vi "TEST - Remove Typedefs from Variant.vi"(8 "error in (no error)":errorcluster) -> (0 "error out":errorcluster, 2 "pass":bool)   [LabVIEW 2020, in "test_openg_variant.lvlib"]
uses:
  test_openg_variant.lvlib
  <userlib>/_OpenG.lib/error/error.llb/openg_error.lvlib
  source/library/openg_variant.lvlib
  Type Def.ctl
panel:
  out "Failures":T1(array[cluster])
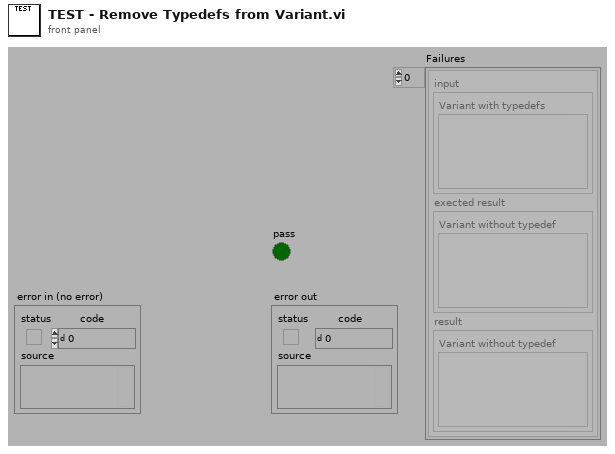
[diagram p1: front panel]
types:
  T1 = cluster{"input":cluster{"Variant with typedefs":variant}, "exected result":cluster{"Variant without typedef":variant}, "result":cluster{"Variant without typedef":variant}}[]
  T2 = typedef "test_openg_variant.lvlib/Type Def.ctl" = dbl
  T3 = cluster{"input":cluster{"Variant with typedefs":variant}, "exected result":cluster{"Variant without typedef":variant}, "result":cluster{"Variant without typedef":variant}}
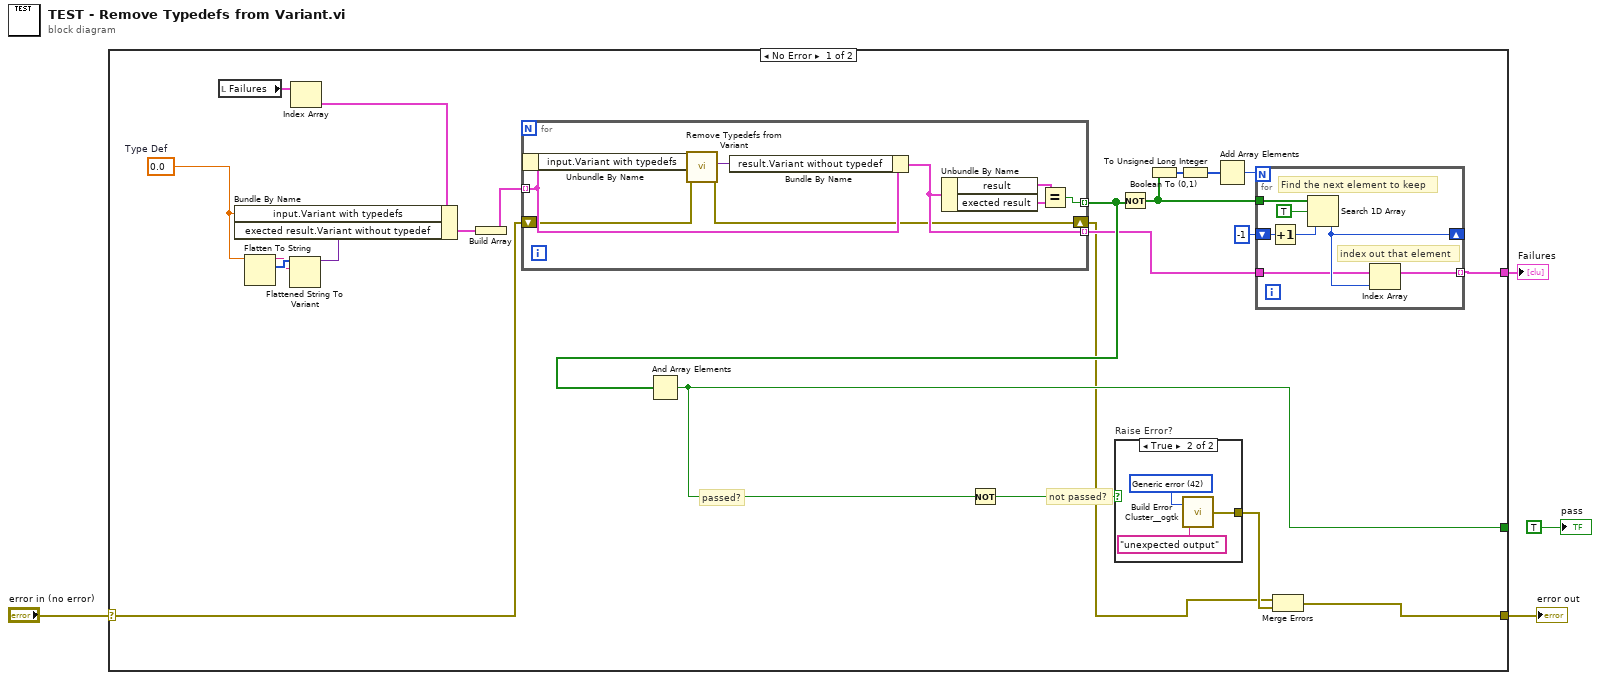
[diagram p0: block diagram]
diagram:
  n1 = case shown="No Error" "error in (no error)" {
    selector: "error in (no error)" -> [w12 w46]
    tunnel: [w23 _] -> _
    tunnel: [w26 w46] -> w3
    tunnel: [w15 _] -> w2
    frame No Error {
      w8 = T2 0.0  # Type Def
      # "not passed?"
      # "passed?"
      n2 = local read "Failures"() -> (w10:T1)
      n3 = Flatten To String(anything=w8) -> (data string=w6:string, type string=w7:i16[])  [unwired: 3 in, 1 out]
      n4 = Flattened String To Variant(6:w6, 7:w7) -> (3:w5:variant)  [unwired: 1 in, 1 out]
      n5 = Index Array(array=w10) -> (element=w9:T3)  [unwired: 1 in]
      n6 = Bundle By Name(cluster=w9, "input.Variant with typedefs"=w8, "exected result.Variant without typedef"=w5) -> (w14:T3)
      n7 = Build Array(w14) -> (w13:T1)
      n8 = for {
        tunnel: w13 -> [w41] mode=indexing
        tunnel: [w42] -> w17 mode=indexing
        tunnel: [w40] -> w16 mode=indexing
        shift-right: [w36] -> w11
        shift-left: w12 -> [w35]
        n9 = Unbundle By Name(w41) -> ("input.Variant with typedefs"=w37:variant)
        n10 = call "Remove Typedefs from Variant.vi"("error in"=w35, "Variant with typedefs"=w37) -> ("error out"=w36:errorcluster, "Variant without typedef"=w34:variant)  [unwired: 8 in]
        n11 = Bundle By Name(cluster=w41, "result.Variant without typedef"=w34) -> (w40:T3)
        n12 = Unbundle By Name(w40) -> ("result"=w39:cluster{"Variant without typedef":variant}, "exected result"=w38:cluster{"Variant without typedef":variant})
        n13 = Equal?(x=w39, y=w38) -> (x = y?=w42:bool)
      }
      n14 = And Array Elements(Boolean array=w17) -> (logical AND=w23:bool)
      n15 = Not(x=w23) -> (.not. x?=w24:bool)
      n16 = case "Raise Error?" shown="True" w24 {
        tunnel: [_ w43] -> w25
        frame False {
        }
        frame True {
          w44 = 42 items=["No error", "Argument error", "Memory is full", "Out of zone", "End of file", "File already open", "Generic file I/O error", "File not found", "File permission error", "Disk is full", "Duplicate path", "Too many files open", "System feature not enabled", "Resource file not found", "Cannot add resource", "Resource not found", "Image not found", "Image memory error", "Pen does not exist", "Config type invalid", "Config token not found", "Config parse error", "Config memory error", "Bad external code format", "Bad external code offset", "External code not present", "Null window", "Destroy window error", "Null menu", "Print aborted", "Bad print record", "Print driver error", "Windows error during printing", "Memory error during printing", "Print dialog error", "Generic print error", "Invalid device refnum", "Device not found", "Device parameter error", "Device unit error", "Cannot open device", "Device call aborted", "Generic error", "Cancelled by user", "Object ID too low", "Object ID too high", "Object not in heap", "Unknown heap", "Unknown object (invalid DefProc)", "Unknown object (DefProc not in table)", "Message out of range", "Invalid (null) method", "Unknown message", "Manager call not supported", "Bad address", "Network operation in progress", "Network operation timed out", "Connection is busy", "Network attribute not supported", "Network error", "Address in use", "System out of memory", "Connection aborted", "Connection refused", "Not connected", "Already connected", "Connection closed", "Initialization error (interapplication manager)", "Bad occurrence", "Wait on unbound occurrence handler", "Occurrence queue overflow", "Datalog type conflict", "Unused", "Unrecognized type (interapplication manager)", "Memory corrupt", "Failed to make temporary DLL", "Old CIN version", "Drag socket not found", "Failed to load drop-object", "Failed to register OLE object", "Failed to release OLE object", "Format specifier type mismatch", "Unknown format specifier", "Too few format specifiers", "Too many format specifiers", "Scan failed", "Newer CIN version", "Error converting to variant", "Runtime menu error", "Password tampered", "Variant attribute not found", "Incompatible variant data type", "Event data is not available", "Event Store is not present", "Occurrence is not found", "Event Queue is not created", "Event info is not available", "Refnum passed is NULL", "Error retrieving Class GUID", "Error retrieving CoClass GUID", "Error retrieving TypeLib GUID.", "Bad built application magic bytes.", "Specific driver is different from the specific driver associated with the Logical Name.", "There is no session opened to the class driver.", "Max Error", "MAX - Error with config objects", "MAX - Error loading configuration", "MAX - Group not supported"]
          n17 = call <userlib>:"Build Error Cluster__ogtk.vi"("String to Prepend to source (\"\")"="unexpected output" ("String to Prepend to source (\"\")"), "code"=w44) -> ("error out"=w43:errorcluster)
        }
      }
      n18 = Not(x=w17) -> (.not. x?=w19:bool[])
      n19 = Boolean To (0,1)(Boolean=w19) -> (0, 1=w20:i16[])
      n20 = To Unsigned Long Integer(number=w20) -> (unsigned 32bit integer=w18:u32[])
      n21 = Add Array Elements(numeric array=w18) -> (sum=w21:u32)
      n22 = for {
        N: w21 -> [_]
        tunnel: w16 -> [w29]
        tunnel: w19 -> [w33]
        shift-right: [w30] -> _
        shift-left: -1 ("start index (0)") -> [w31]
        tunnel: [w28] -> w15 mode=indexing
        # "index out that element"
        # "Find the next element to keep"
        n23 = Increment(x=w31) -> (x+1=w27:i32)
        n24 = Search 1D Array(1D array=w33, element=TRUE, start index (0)=w27) -> (index of element=w30:i32)
        n25 = Index Array(array=w29, index=w30) -> (element=w28:T3)
      }
      n26 = Merge Errors(w11, w25) -> (w26:errorcluster)
    }
    frame Error {
    }
  }
  "error out" <- w3
  "Failures" <- w2
  "pass" <- TRUE ("pass")
